vi "Acquire T1 Waveform.vi"(8 "error in":errorcluster, 11 "sampling frequency":dbl=98816000.0 format="%#.2p") -> (0 "error out":errorcluster, 3 "Waveform":waveform(dbl))   [LabVIEW 2018]
doc: "Generate a simulated T1 signal based on an input frequency."
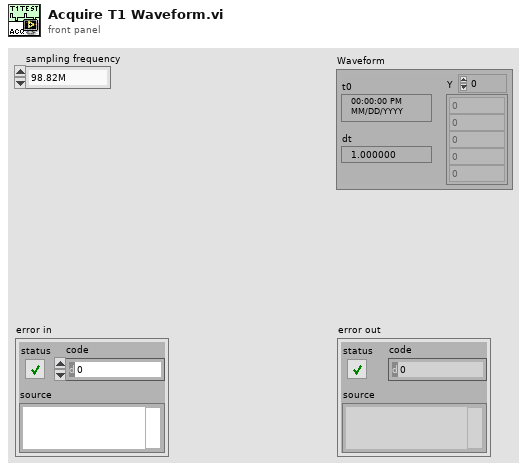
[diagram p1: front panel]
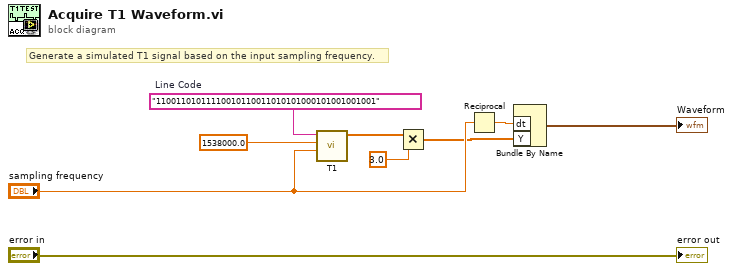
[diagram p0: block diagram]
diagram:
  w7 = "11001101011110010110011010101000101001001001"  # Line Code
  # "Generate a simulated T1 signal based on the input sampling frequency."
  n1 = call "T1.vi"("Sampling Frequency"="sampling frequency", "Frequency"=1538000.0, "Line Code"=w7) -> ("Binary Waveform"=w5:dbl[])  [unwired: 7 in, 1 out]
  n2 = Multiply(x=w5, y=3.0) -> (x*y=w4:dbl[])
  n3 = Reciprocal(x="sampling frequency") -> (1/x=w6:dbl)
  n4 = Bundle By Name("dt"=w6, "Y"=w4) -> (→"Waveform":waveform(dbl))  [unwired: 1 in]
  "error out" <- "error in"
